vi "Leitura de dados txt.vi"() -> ()   [LabVIEW 2014]
uses:
  leitura de dados txt control.ctl
  <vilib>/Utility/file.llb/Read From Spreadsheet File (string).vi
panel:
  out "XY Graph":cluster{"X":dbl, "Y":dbl}[](graph)
  out "NeedInterpolation?":bool
  out "Collumns":i32
  out "Rows":i32
  out "all rows":string[][](array[string])
  out "Matrix collumn Index":dbl
  in  "Iluminantes":T1
  # "Selecione o iluminante que deseja utilizar."
  # "Indicadores de testes"
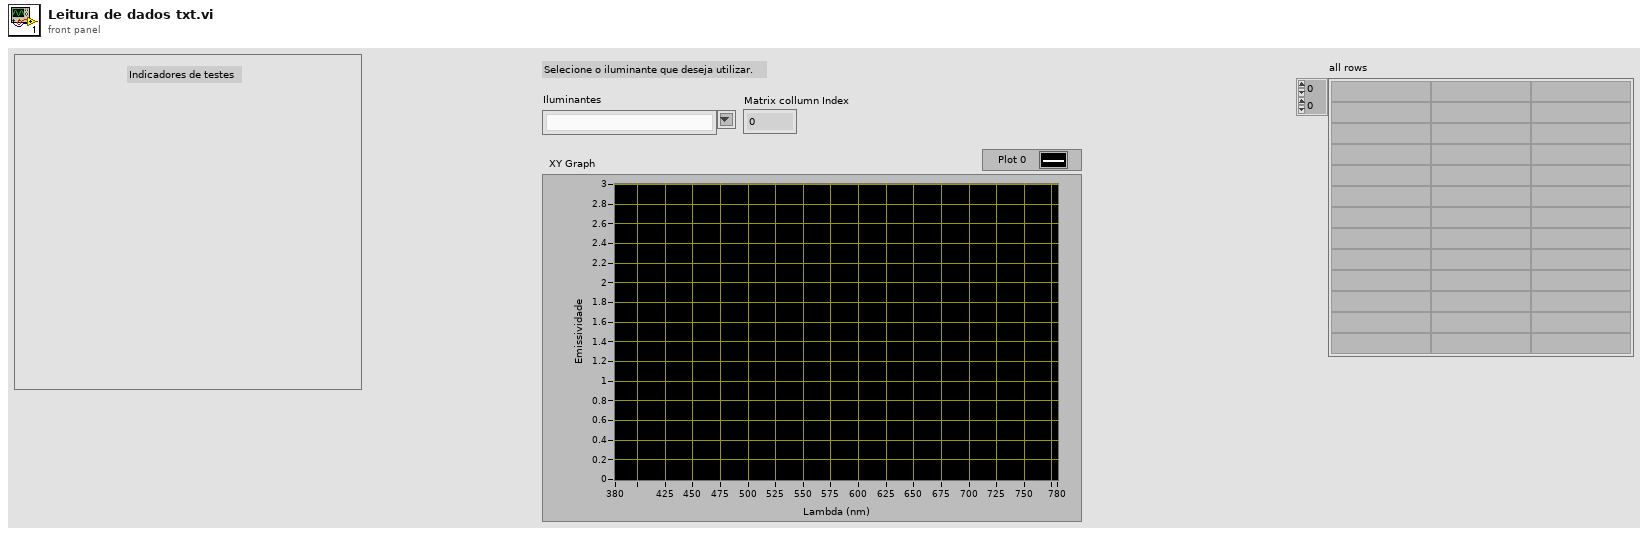
[diagram p1: front panel]
types:
  T1 = typedef "leitura de dados txt control.ctl" = string
  T2 = typedef "Control 1" = string
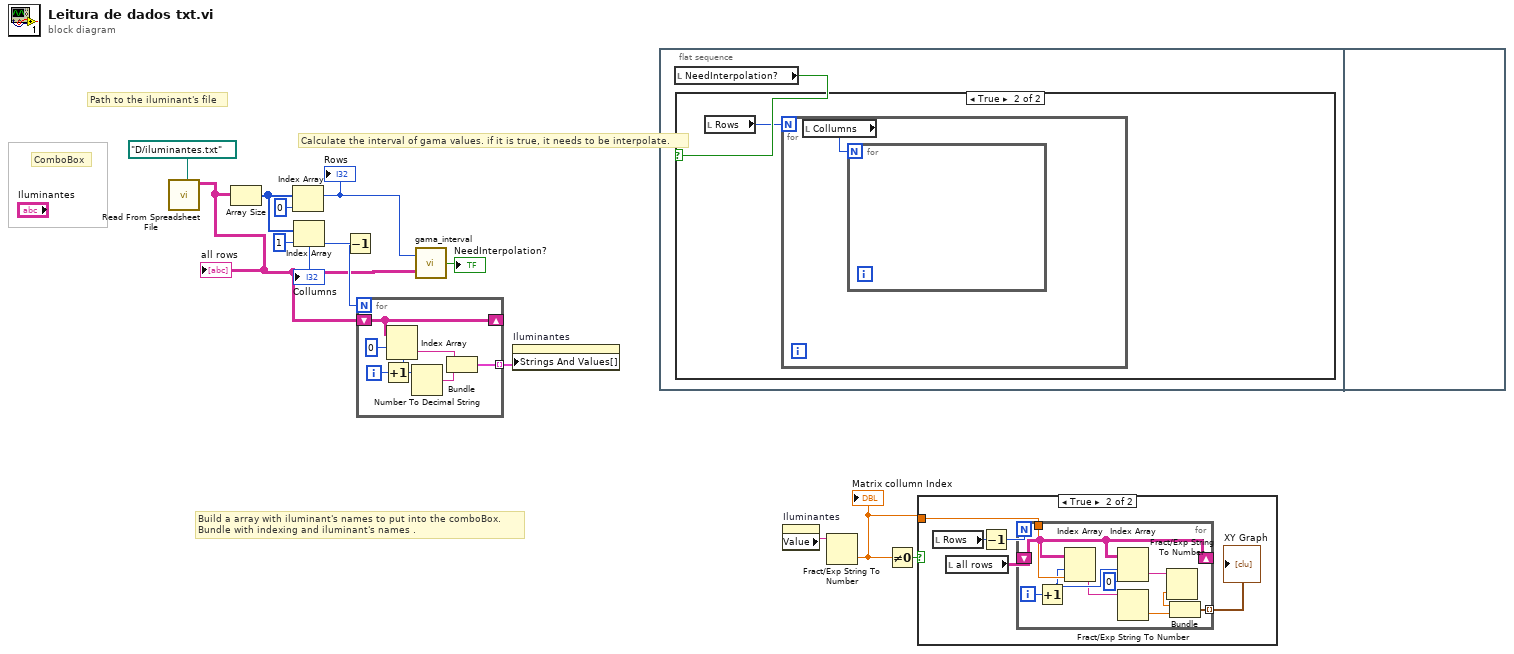
[diagram p0: block diagram]
diagram:
  # "Calculate the interval of gama values. if it is true, it needs to be interpolate."
  # "Path to the iluminant's file"
  # "ComboBox"
  # "Build a array with iluminant's names to put into the comboBox.\nBundle with indexing and iluminant's names ."
  n1 = call-poly <vilib>:"Read From Spreadsheet File.vi"("file path (dialog if empty)"=path "D:/iluminantes.txt") -> ("all rows"=w5:string[][])  [unwired: 6 in, 4 out]
  "all rows" <- w5
  n2 = Array Size(array=w5) -> (size(s)=w11:i32[])
  n3 = Index Array(array=w11, index=0) -> (element=w6:i32)
  "Rows" <- w6
  n4 = Index Array(array=w11, index=1) -> (element=w9:i32)
  "Collumns" <- w9
  n5 = Decrement(x=w9) -> (x-1=w8:i32)
  n6 = for {
    N: w8 -> [_]
    shift-right: [w18] -> _
    shift-left: w5 -> [w18]
    tunnel: [w14] -> w7 mode=indexing
    i -> [w20]
    n7 = Increment(x=w20) -> (x+1=w17:i32)
    n8 = Index Array(array=w18, index (row)=0, index (col)=w17) -> (element=w15:string)
    n9 = Number To Decimal String(number=w17) -> (decimal integer string=w16:string)  [unwired: 1 in]
    n10 = Bundle("String"=w15, w16) -> (w14:cluster{"String":string, string})  [unwired: 1 in]
  }
  n11 = call "gama_interval.vi"("Matrix with txt"=w5, "Number of Rows"=w6) -> ("isNotFive?"=→"NeedInterpolation?":bool)
  n12 = property on="Iluminantes" class="CmbBox (strict)"("Strings And Values[]"=w7) -> ()  [unwired: 2 in, 2 out]
  n13 = flat-sequence {
    frame #0 {
      n14 = local read "NeedInterpolation?"() -> (w21:bool)
      n15 = case shown="True" w21 {
        frame False {
        }
        frame True {
          n16 = local read "Rows"() -> (w22:i32)
          n17 = for {
            N: w22 -> [_]
            n18 = local read "Collumns"() -> (w23:i32)
            n19 = for {
              N: w23 -> [_]
            }
          }
        }
      }
    }
    frame #1 {
    }
  }
  n20 = property on="Iluminantes" class="CmbBox (strict)"() -> ("Value"=w3:T2)  [unwired: 2 in, 2 out]
  n21 = Fract/Exp String To Number(string=w3) -> (number=w1:dbl)  [unwired: 3 in, 1 out]
  "Matrix collumn Index" <- w1
  n22 = Not Equal To 0?(x=w1) -> (x != 0?=w2:bool)
  n23 = case shown="True" w2 {
    tunnel: w1 -> [_ w24]
    frame False {
    }
    frame True {
      n24 = local read "Rows"() -> (w27:i32)
      n25 = local read "all rows"() -> (w26:string[][])
      n26 = Decrement(x=w27) -> (x-1=w28:i32)
      n27 = for {
        N: w28 -> [_]
        shift-right: [w36] -> _
        shift-left: w26 -> [w36]
        tunnel: w24 -> [w37]
        tunnel: [w33] -> w25 mode=indexing
        i -> [w38]
        n28 = Increment(x=w38) -> (x+1=w35:i32)
        n29 = Index Array(array=w36, index (row)=w35, index (col)=w37) -> (element=w31:string)
        n30 = Index Array(array=w36, index (row)=w35, index (col)=0 ("disabled index (col)")) -> (element=w32:string)
        n31 = Fract/Exp String To Number(string=w31) -> (number=w29:dbl)  [unwired: 3 in, 1 out]
        n32 = Fract/Exp String To Number(string=w32) -> (number=w30:dbl)  [unwired: 3 in, 1 out]
        n33 = Bundle(w30, w29) -> (w33:cluster{dbl, dbl})  [unwired: 1 in]
      }
      "XY Graph" <- w25
    }
  }
